vi "example - MsgQ.vi"() -> ()   [LabVIEW 2016, in "MsgQ.lvlib"]
uses:
  MsgQ.lvlib
panel:
  out "# iterations":i32
  out "NotifArray":string[](array[string])
  out "MsgQ tout":bool
  out "timed out?":bool
  out "Response Code":dbl
  out "Response":string[](array[string])
  out "error out":errorcluster
  in  "Data2":string[](array[string])=["four", "five"]
  in  "Data1":string[](array[string])=["one", "two", "three"]
  out "Data out":string[](array[string])
  in  "stop":bool
  in  "Send2":bool
  in  "Send1":bool
  # "Response"
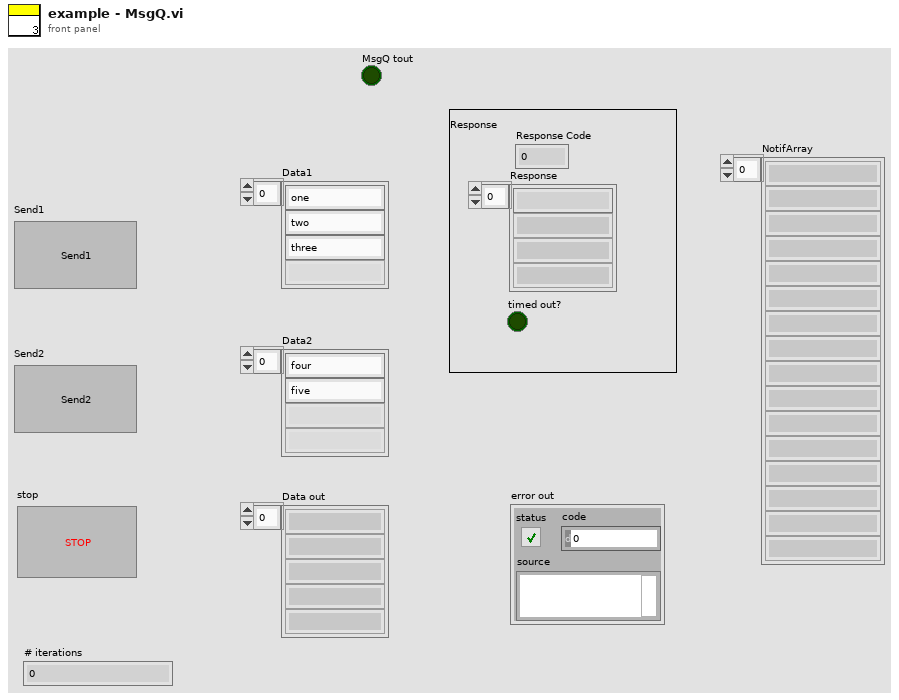
[diagram p1: front panel]
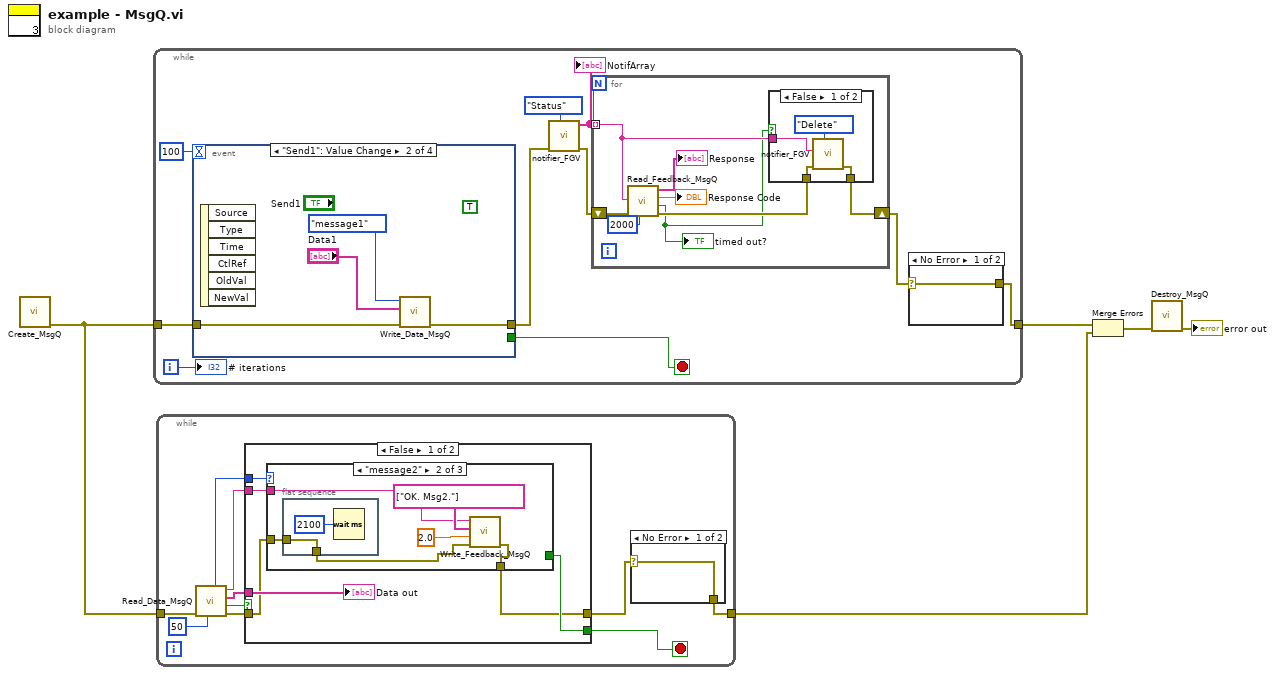
[diagram p0: block diagram]
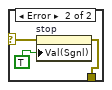
[diagram p2: hidden frame]
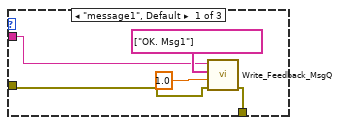
[diagram p3: hidden frame]
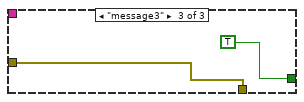
[diagram p4: hidden frame]
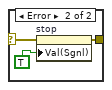
[diagram p7: hidden frame]
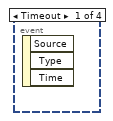
[diagram p8: hidden frame]
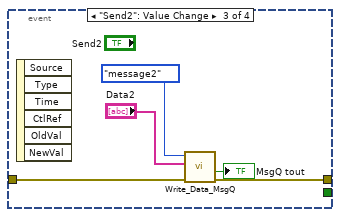
[diagram p9: hidden frame]
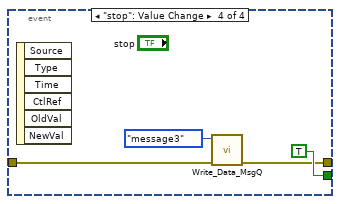
[diagram p10: hidden frame]
diagram:
  n1 = call "Create_MsgQ.vi"() -> ("error out"=w5:errorcluster)  [unwired: 10 in, 1 out]
  n2 = while {
    tunnel: w5 -> [w13]
    tunnel: [w12] -> w4
    i -> [w6]
    stop <- w14 stop-if-true
    n3 = event shown="[1] \"Send1\": Value Change" {
      selector: _ -> [_ _ _ _]
      dyn-events: _ -> [_ _ _ _]
      timeout: 100 -> [_ _ _ _]
      tunnel: [_ _ _ TRUE] -> w14
      tunnel: w13 -> [_ w36 w40 w43]
      tunnel: [_ w35 w39 w42] -> w9
      event Timeout {
        n4 = event-data() -> ()  [unwired: 1 in, 3 out]
      }
      event "Send1": Value Change {
        (unwired) TRUE
        n5 = event-data() -> ()  [unwired: 1 in, 6 out]
        n6 = call "Write_Data_MsgQ.vi"("error in (no error)"=w36, "Data in"="Data1", "Command"=enum16{"message1", "message2", "message3"}."message1") -> ("error out"=w35:errorcluster)  [unwired: 6 in, 2 out]
      }
      event "Send2": Value Change {
        n7 = event-data() -> ()  [unwired: 1 in, 6 out]
        n8 = call "Write_Data_MsgQ.vi"("error in (no error)"=w40, "Data in"="Data2", "Command"=enum16{"message1", "message2", "message3"}."message2") -> ("error out"=w39:errorcluster, "timed out?"=→"MsgQ tout":bool)  [unwired: 6 in, 1 out]
      }
      event "stop": Value Change {
        n9 = event-data() -> ()  [unwired: 1 in, 6 out]
        n10 = call "Write_Data_MsgQ.vi"("error in (no error)"=w43, "Command"=enum16{"message1", "message2", "message3"}."message3") -> ("error out"=w42:errorcluster)  [unwired: 7 in, 2 out]
      }
    }
    n11 = call "notifier_FGV.vi"("Mode"=enum16{"Status", "Add", "Access", "Delete"}."Status", "error in (no error)"=w9) -> ("error out"=w8:errorcluster, "NotifArray"=w10:string[])  [unwired: 6 in, 2 out]
    "NotifArray" <- w10
    n12 = for {
      shift-right: [w18] -> w11
      shift-left: w8 -> [w21]
      tunnel: w10 -> [w19] mode=indexing
      n13 = call "Read_Feedback_MsgQ.vi"("timeout in ms (2000)"=2000, "error in (no error)"=w21, "ResponseAddr in"=w19) -> ("error out"=w20:errorcluster, "timed out?"=w17:bool, "Code"=→"Response Code":dbl, "Data out"=→"Response":string[])  [unwired: 5 in]
      "timed out?" <- w17
      n14 = case shown="False" w17 {
        tunnel: w20 -> [w27 w28]
        tunnel: w19 -> [w25 _]
        tunnel: [w24 w28] -> w18
        frame False {
          n15 = call "notifier_FGV.vi"("Mode"=enum16{"Status", "Add", "Access", "Delete"}."Delete", "error in (no error)"=w27, "ResponseAddr in"=w25) -> ("error out"=w24:errorcluster)  [unwired: 5 in, 3 out]
        }
        frame True {
        }
      }
    }
    n16 = case shown="No Error" w11 {
      selector: w11 -> [w29 w32]
      tunnel: [w29 w30] -> w12
      frame No Error {
      }
      frame Error {
        n17 = property on="stop" class="Bool (strict)"(error in=w32, "Val(Sgnl)"=TRUE) -> (error out=w30:errorcluster)  [unwired: 1 in, 1 out]
      }
    }
    "# iterations" <- w6
  }
  n18 = while {
    tunnel: w5 -> [w55]
    tunnel: [w48] -> w3
    stop <- w50 stop-if-true
    n19 = call "Read_Data_MsgQ.vi"("timeout in ms (10)"=50, "error in (no error)"=w55) -> ("error out"=w52:errorcluster, "timed out?"=w53:bool, "Data out"=w51:string[], "ResponseAddr"=w46:string, "Command out"=w47:enum16{"message1", "message2", "message3"})  [unwired: 5 in]
    n20 = case shown="False" w53 {
      tunnel: w52 -> [w61 w81]
      tunnel: w51 -> [w65 _]
      tunnel: w47 -> [w64 _]
      tunnel: [w63 _] -> w50
      tunnel: [w62 w81] -> w49
      tunnel: w46 -> [w60 _]
      frame False {
        n21 = case shown="\"message2\"" w64 {
          tunnel: [_ _ TRUE] -> w63
          tunnel: [w70 w74 w79] -> w62
          tunnel: w61 -> [w67 w73 w79]
          tunnel: w60 -> [w66 w71 _]
          frame "message1", Default {
            n22 = call "Write_Feedback_MsgQ.vi"("error in (no error)"=w67, "Code"=1.0, "Data in"=string[] ["OK. Msg1"], "ResponseAddr"=w66) -> ("error out"=w70:errorcluster)  [unwired: 7 in]
          }
          frame "message2" {
            n23 = flat-sequence {
              tunnel: w73 -> [w77]
              tunnel: [w77] -> w72
              frame #0 {
                n24 = Wait (ms)(milliseconds to wait=u32 2100) -> ()  [unwired: 1 out]
              }
            }
            n25 = call "Write_Feedback_MsgQ.vi"("error in (no error)"=w72, "Code"=2.0, "Data in"=string[] ["OK. Msg2."], "ResponseAddr"=w71) -> ("error out"=w74:errorcluster)  [unwired: 7 in]
          }
          frame "message3" {
          }
        }
        "Data out" <- w65
      }
      frame True {
      }
    }
    n26 = case shown="No Error" w49 {
      selector: w49 -> [w56 w59]
      tunnel: [w56 w57] -> w48
      frame No Error {
      }
      frame Error {
        n27 = property on="stop" class="Bool (strict)"(error in=w59, "Val(Sgnl)"=TRUE) -> (error out=w57:errorcluster)  [unwired: 1 in, 1 out]
      }
    }
  }
  n28 = Merge Errors(w4, w3) -> (w2:errorcluster)
  n29 = call "Destroy_MsgQ.vi"("error in (no error)"=w2) -> ("error out"=→"error out":errorcluster)  [unwired: 10 in]
